vi "One Step Normalized.vi"(6 "eps":dbl, 9 "table":dbl[][](array[numeric]) format="%.1f", 10 "n-m":u32[](array[numeric]), 11 "m":u32[](array[numeric])) -> (0 "error":i32, 1 "table*":dbl[][](array[numeric]) format="%.1f", 2 "n-m*":u32[](array[numeric]), 3 "m*":u32[](array[numeric]))   [LabVIEW 2020, in "NI_Gmath.lvlib"]
uses:
  <vilib>/gmath/NI_Gmath.lvlib
  <vilib>/Analysis/NI_AALBLAS.lvlib
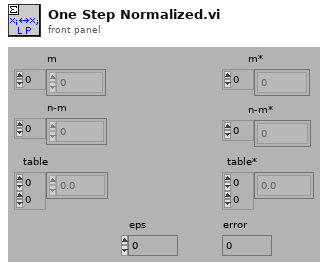
[diagram p1: front panel]
types:
  T1 = typedef "NI_Matrix.lvlib/RealMatrix.ctl" = dbl[][]
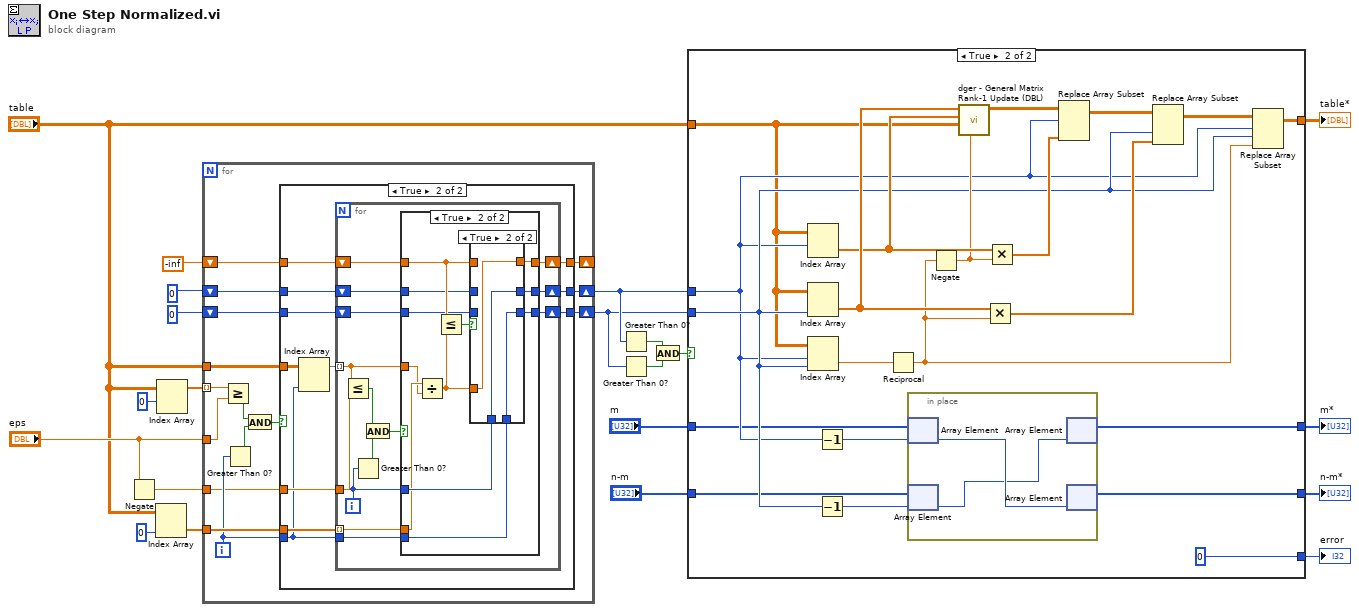
[diagram p0: block diagram]
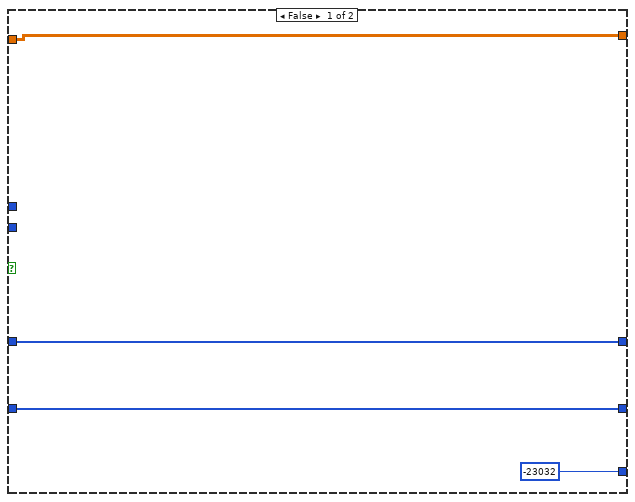
[diagram p2: hidden frame]
diagram:
  n1 = Negate(x="eps") -> (-x=w5:dbl)
  n2 = Index Array(array="table", index (col)=0) -> (element=w7:dbl[])  [unwired: 1 in]
  n3 = Index Array(array="table", index (row)=0) -> (element=w11:dbl[])  [unwired: 1 in]
  n4 = for {
    tunnel: w11 -> [w24] mode=indexing
    tunnel: "table" -> [w26]
    shift-right: [w31] -> w3
    shift-left: 0 -> [w32]
    shift-right: [w29] -> w2
    shift-left: 0 -> [w30]
    tunnel: w7 -> [w33]
    shift-right: [w27] -> _
    shift-left: -inf -> [w28]
    tunnel: "eps" -> [w23]
    tunnel: w5 -> [w22]
    i -> [w25]
    n5 = Greater Or Equal?(x=w24, y=w23) -> (x >= y?=w35:bool)
    n6 = Greater Than 0?(x=w25) -> (x > 0?=w36:bool)
    n7 = And(x=w35, y=w36) -> (x .and. y?=w34:bool)
    n8 = case shown="True" w34 {
      tunnel: w26 -> [_ w42]
      tunnel: w33 -> [_ w50]
      tunnel: w32 -> [w39 w49]
      tunnel: [w39 w47] -> w31
      tunnel: w30 -> [w38 w48]
      tunnel: [w38 w46] -> w29
      tunnel: w28 -> [w37 w45]
      tunnel: [w37 w44] -> w27
      tunnel: w25 -> [_ w40]
      tunnel: w22 -> [_ w41]
      frame False {
      }
      frame True {
        n9 = Index Array(array=w42, index (col)=w40) -> (element=w43:dbl[])  [unwired: 1 in]
        n10 = for {
          tunnel: w43 -> [w52] mode=indexing
          tunnel: w50 -> [w61] mode=indexing
          shift-right: [w59] -> w47
          shift-left: w49 -> [w60]
          shift-right: [w57] -> w46
          shift-left: w48 -> [w58]
          shift-right: [w55] -> w44
          shift-left: w45 -> [w56]
          tunnel: w40 -> [w53]
          tunnel: w41 -> [w51]
          i -> [w54]
          n11 = Less Or Equal?(x=w52, y=w51) -> (x <= y?=w63:bool)
          n12 = Greater Than 0?(x=w54) -> (x > 0?=w64:bool)
          n13 = And(x=w63, y=w64) -> (x .and. y?=w62:bool)
          n14 = case shown="True" w62 {
            tunnel: w52 -> [_ w69]
            tunnel: w61 -> [_ w70]
            tunnel: w60 -> [w67 w72]
            tunnel: [w67 w77] -> w59
            tunnel: w58 -> [w66 w71]
            tunnel: [w66 w75] -> w57
            tunnel: w56 -> [w65 w73]
            tunnel: [w65 w74] -> w55
            tunnel: w54 -> [_ w78]
            tunnel: w53 -> [_ w76]
            frame False {
            }
            frame True {
              n15 = Divide(x=w70, y=w69) -> (x/y=w68:dbl)
              n16 = Less Or Equal?(x=w73, y=w68) -> (x <= y?=w79:bool)
              n17 = case shown="True" w79 {
                tunnel: w78 -> [_ w85]
                tunnel: [w81 w85] -> w77
                tunnel: w76 -> [_ w84]
                tunnel: [w80 w84] -> w75
                tunnel: [w82 w83] -> w74
                tunnel: w68 -> [_ w83]
                tunnel: w73 -> [w82 _]
                tunnel: w72 -> [w81 _]
                tunnel: w71 -> [w80 _]
                frame False {
                }
                frame True {
                }
              }
            }
          }
        }
      }
    }
  }
  n18 = Greater Than 0?(x=w3) -> (x > 0?=w21:bool)
  n19 = Greater Than 0?(x=w2) -> (x > 0?=w20:bool)
  n20 = And(x=w21, y=w20) -> (x .and. y?=w4:bool)
  n21 = case shown="True" w4 {
    tunnel: w2 -> [_ w100]
    tunnel: w3 -> [_ w99]
    tunnel: [w86 w98] -> w18
    tunnel: "m" -> [w88 w97]
    tunnel: [w88 w96] -> w16
    tunnel: "n-m" -> [w87 w95]
    tunnel: [w87 w94] -> w14
    tunnel: "table" -> [w86 w91]
    tunnel: [-23032 0] -> w1
    frame False {
    }
    frame True {
      n22 = Index Array(array=w91, index (row)=w99) -> (element=w104:dbl[])  [unwired: 1 in]
      n23 = Index Array(array=w91, index (col)=w100) -> (element=w105:dbl[])  [unwired: 1 in]
      n24 = Index Array(array=w91, index (row)=w99, index (col)=w100) -> (element=w108:dbl)
      n25 = Decrement(x=w99) -> (x-1=w93:i32)
      n26 = Decrement(x=w100) -> (x-1=w92:i32)
      n27 = Reciprocal(x=w108) -> (1/x=w101:dbl)
      n28 = in-place {
        n29 = in-place-array #1(w97, w93) -> (w112:u32)
        n30 = in-place-array #2(w95, w92) -> (w111:u32)
        n31 = in-place-array #1(w111) -> (w96:u32[])  [unwired: 1 out]
        n32 = in-place-array #2(w112) -> (w94:u32[])  [unwired: 1 out]
      }
      n33 = Negate(x=w101) -> (-x=w102:dbl)
      n34 = call <vilib>:"dger - General Matrix Rank-1 Update (DBL).vi"("alpha"=w102, "A"=w91, "y"=w104, "x"=w105) -> ("dger"=w103:T1)  [unwired: 6 in, 1 out]
      n35 = Multiply(x=w105, y=w101) -> (x*y=w109:dbl[])
      n36 = Multiply(x=w104, y=w102) -> (x*y=w110:dbl[])
      n37 = Replace Array Subset(array=w103, new element=w110, index (row)=w99) -> (w107:T1)  [unwired: 1 in]
      n38 = Replace Array Subset(array=w107, new element=w109, index (col)=w100) -> (w106:T1)  [unwired: 1 in]
      n39 = Replace Array Subset(array=w106, new element=w101, index (row)=w99, index (col)=w100) -> (w98:T1)
    }
  }
  "table*" <- w18
  "n-m*" <- w14
  "m*" <- w16
  "error" <- w1
